vi "Write Selection Visible.vi"(8 "error in (no error)":errorcluster, 10 "Selection Visible":bool=TRUE, 11 "Shape in":refnum<class "Shape.lvclass">) -> (0 "error out":errorcluster, 3 "Shape out":refnum<class "Shape.lvclass">)   [LabVIEW 2015, in "LV Image Editor Framework.lvlib" / "Shape.lvclass"]
uses:
  Shape.lvclass
  Shape.lvclass/Shape.ctl
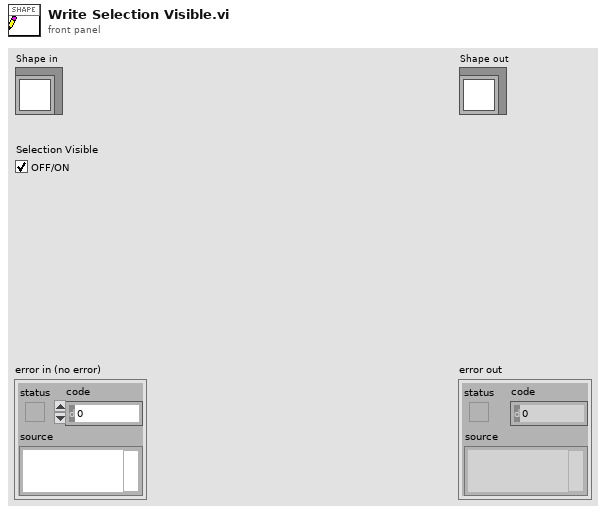
[diagram p1: front panel]
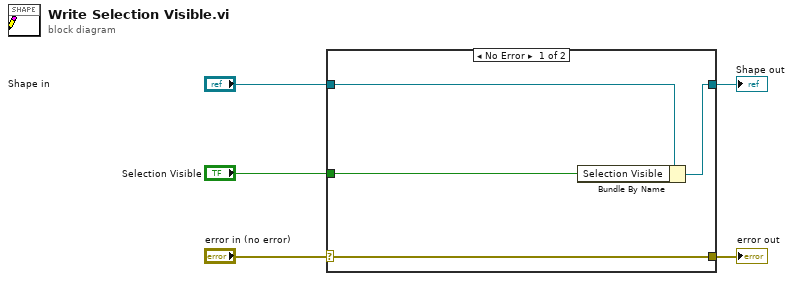
[diagram p0: block diagram]
diagram:
  n1 = case shown="No Error" "error in (no error)" {
    selector: "error in (no error)" -> [w9 w10]
    tunnel: [w9 w10] -> w4
    tunnel: [w7 w11] -> w2
    tunnel: "Shape in" -> [w8 w11]
    tunnel: "Selection Visible" -> [w6 _]
    frame No Error {
      n2 = Bundle By Name(cluster=w8, "Selection Visible"=w6) -> (w7:refnum<class "Shape.lvclass">)
    }
    frame Error {
    }
  }
  "error out" <- w4
  "Shape out" <- w2
